vi "Optical Beacon - Hazardous Area Standard.vi"() -> ()   [LabVIEW 2015]
uses:
  <vilib>/userdefined/High Color/IMAQdx.ctl
  <vilib>/vision/driver/NI_Vision_Acquisition_Software.lvlib
  <vilib>/vision/NI_Vision_Development_Module.lvlib
  <resource>/objmgr/imaqdx.rc
panel:
  in  "Stop 2":bool
  out "Optical Beacon":bool
  out "Color Spectrum 4":dbl[](array[numeric]) format="%.2f"
  in  "Color Sensitivity 4":u32(ring) items=["Low", "Medium", "High"]
  out "Image 4":T1(plugin-control)
  out "Color Spectrum 3":dbl[](array[numeric]) format="%.2f"
  in  "Color Sensitivity 3":u32(ring) items=["Low", "Medium", "High"]
  out "Image 3":T1(plugin-control)
  out "Y Resoloution":i32
  out "X Resoloution":i32
  out "Video Modes":string
  in  "Video Mode":dbl min=0.0 max=5.0 step=1.0
  in  "Camera":T2
  in  "Stop":bool
  out "Image 1":T1(plugin-control)
  in  "Color Sensitivity 1":u32(ring) items=["Low", "Medium", "High"]
  out "Color Spectrum 1":dbl[](array[numeric]) format="%.2f"
  out "YELLOW Close":bool
  out "YELLOW Detect":bool
  out "RED Close":bool
  out "RED Detect":bool
  out "Hazardous Area":bool
  out "Image 2":T1(plugin-control)
  in  "Color Sensitivity 2":u32(ring) items=["Low", "Medium", "High"]
  out "Color Spectrum 2":dbl[](array[numeric]) format="%.2f"
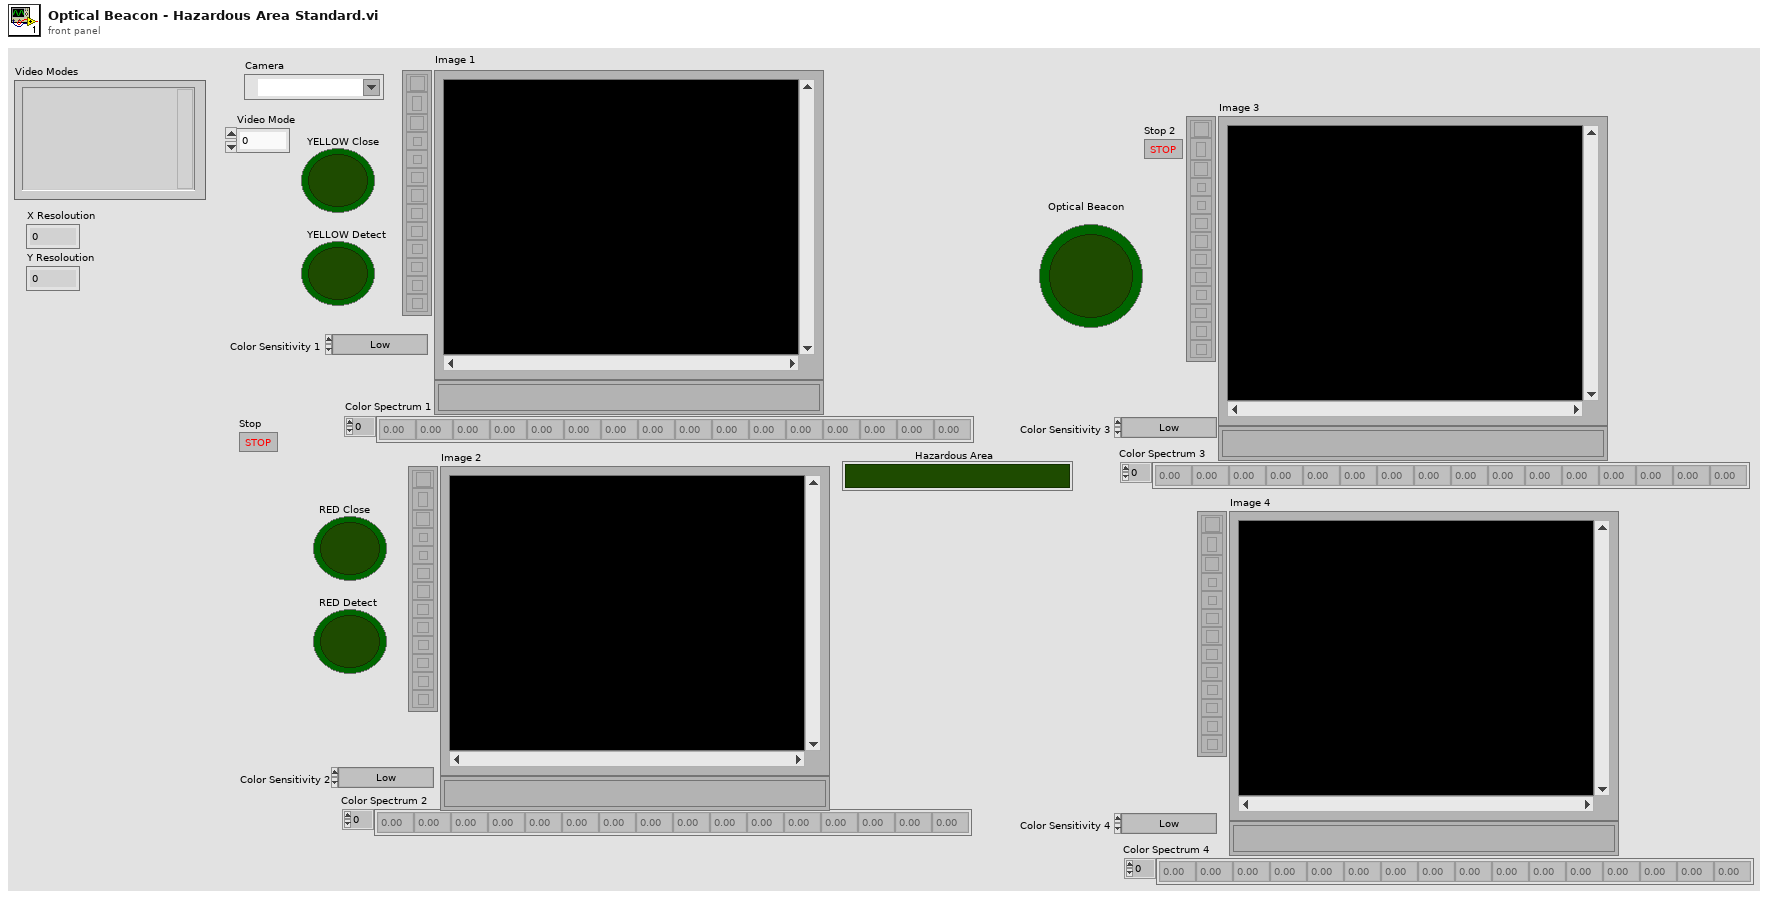
[diagram p1: front panel]
types:
  T1 = typedef "IMAQ Image.ctl" = refnum<image>
  T2 = typedef "IMAQdx.ctl" = refnum<k21>
  T3 = cluster{"Global Rectangle":i32[], "Contours":cluster{"Contour Type":u32, "ROI Type":u32, "Points":i32[]}[]}
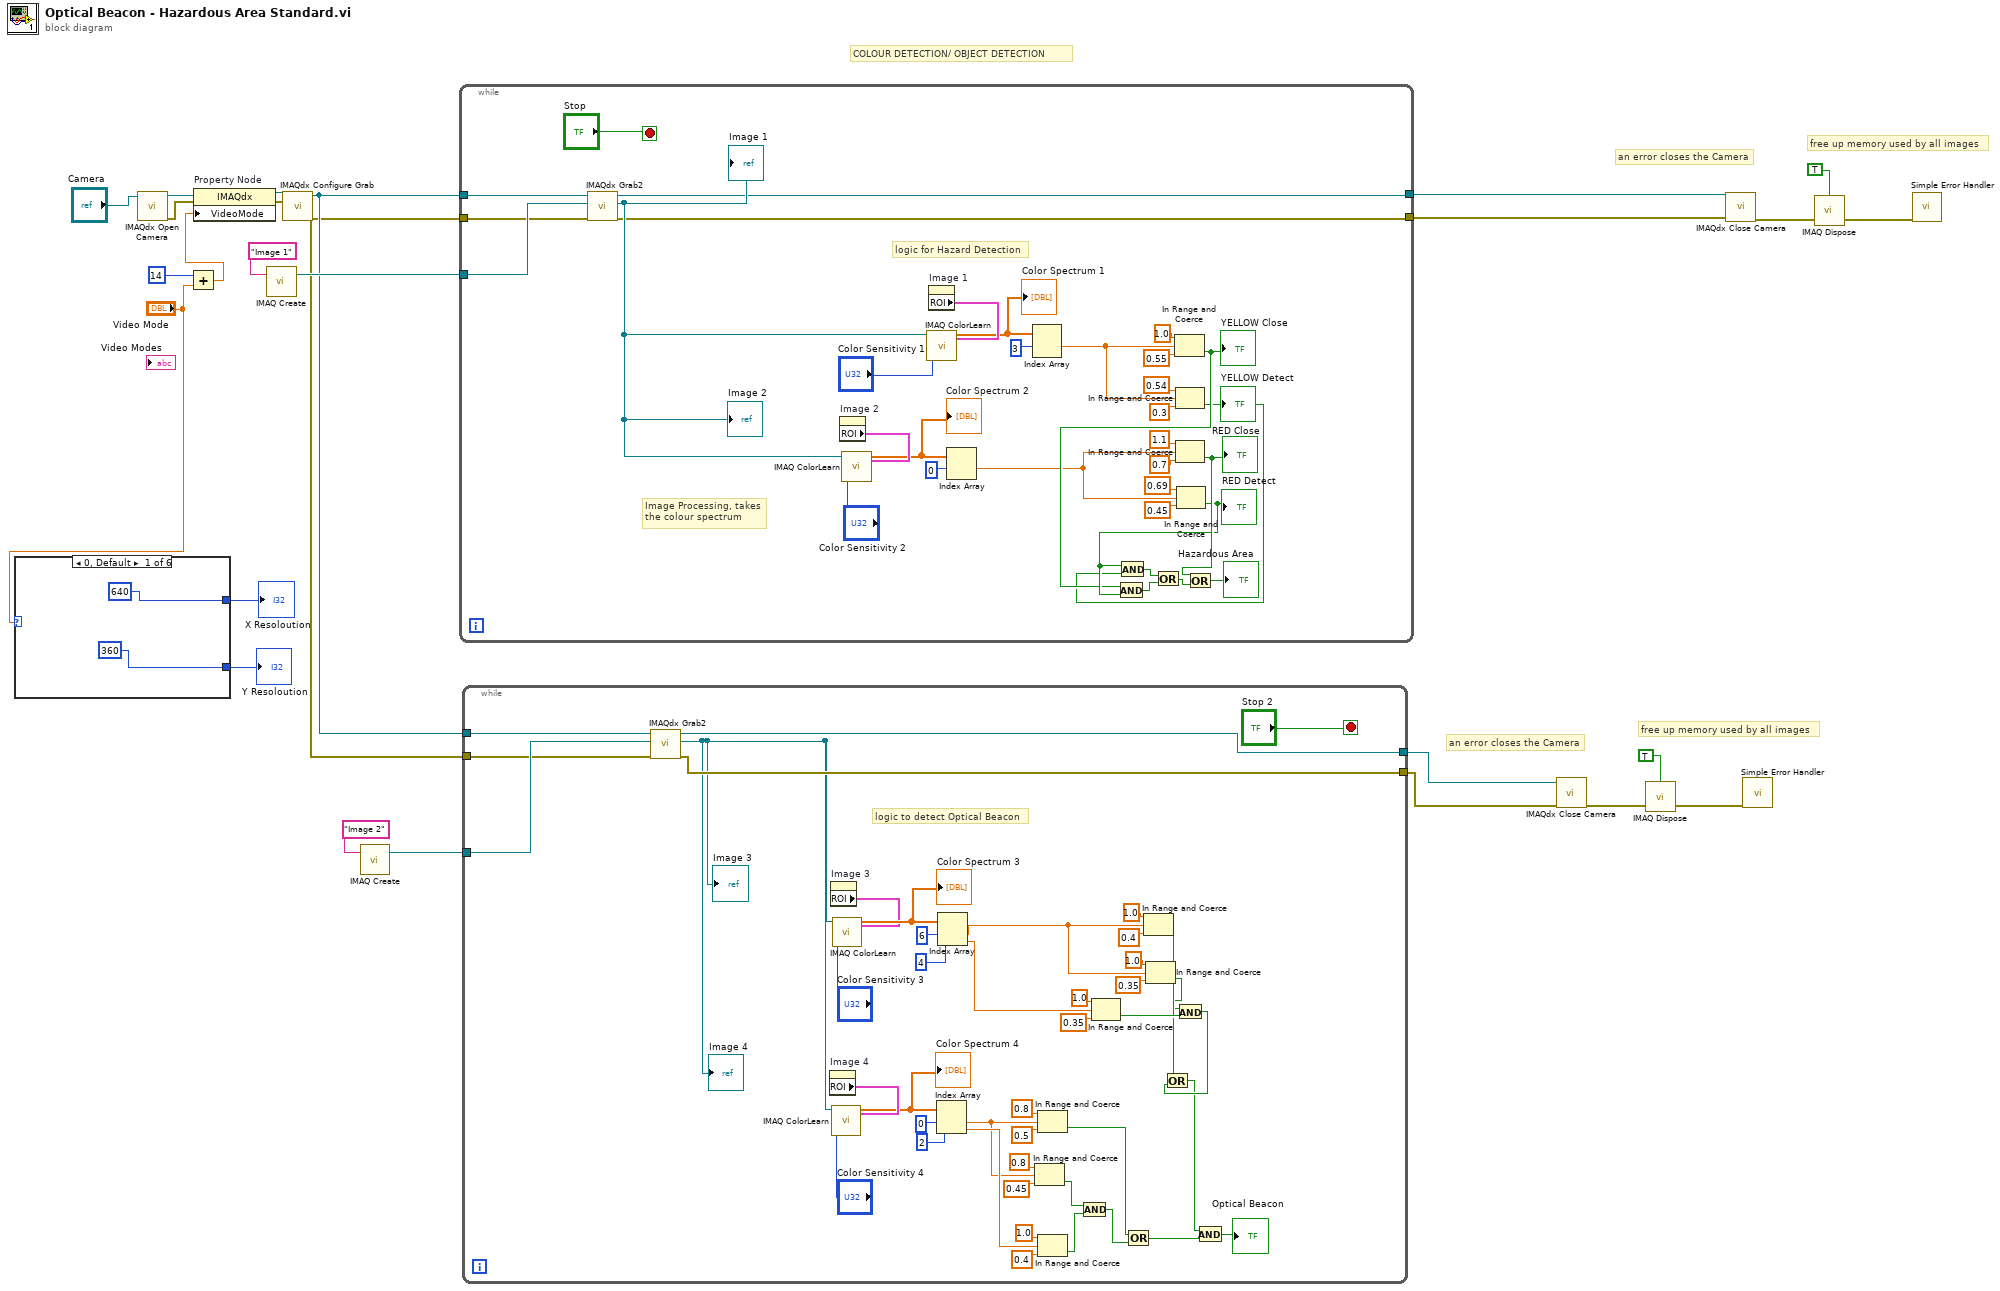
[diagram p0: block diagram]
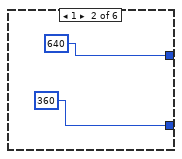
[diagram p2: hidden frame]
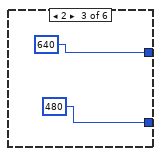
[diagram p3: hidden frame]
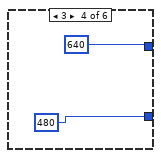
[diagram p4: hidden frame]
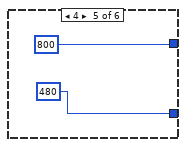
[diagram p5: hidden frame]
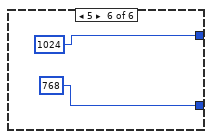
[diagram p6: hidden frame]
diagram:
  # "an error closes the Camera"
  # "free up memory used by all images"
  # "COLOUR DETECTION/ OBJECT DETECTION"
  # "an error closes the Camera"
  # "free up memory used by all images"
  n1 = case shown="0, Default" "Video Mode" {
    tunnel: [640 640 640 640 800 1024] -> w11
    tunnel: [360 360 480 480 480 768] -> w10
    frame 0, Default {
    }
    frame 1 {
    }
    frame 2 {
    }
    frame 3 {
    }
    frame 4 {
    }
    frame 5 {
    }
  }
  "X Resoloution" <- w11
  "Y Resoloution" <- w10
  n2 = call <vilib>:"IMAQdx Open Camera.vi"("Session In"="Camera") -> ("error out"=w23:errorcluster, "Session Out"=w24:T2)  [unwired: 9 in]
  n3 = Add(x=14, y="Video Mode") -> (x+y=w14:dbl)
  n4 = property on="Property Node" class="IMAQdx"(reference=w24, error in=w23, "VideoMode"=w14) -> (reference out=w22:T2, error out=w21:errorcluster)
  n5 = call "IMAQ Create"("Image Name"="Image 1") -> ("New Image"=w25:T1)  [unwired: 4 in, 1 out]
  n6 = call <vilib>:"IMAQdx Configure Grab.vi"("error in"=w21, "Session In"=w22) -> ("error out"=w1:errorcluster, "Session Out"=w2:T2)  [unwired: 8 in]
  n7 = call "IMAQ Create"("Image Name"="Image 2") -> ("New Image"=w3:T1)  [unwired: 4 in, 1 out]
  n8 = while {
    tunnel: w2 -> [w70]
    tunnel: w1 -> [w42]
    tunnel: [w39] -> w13
    tunnel: [w40] -> w19
    tunnel: w25 -> [w69]
    stop <- "Stop" stop-if-true
    # "Image Processing, takes\nthe colour spectrum"
    # "logic for Hazard Detection"
    n9 = call <vilib>:"IMAQdx Grab2.vi"("error in"=w42, "Image In"=w69, "Session In"=w70) -> ("error out"=w40:errorcluster, "Image Out"=w41:T1, "Session Out"=w39:T2)  [unwired: 5 in, 1 out]
    "Image 1" <- w41
    "Image 2" <- w41
    n10 = property on="Image 2" class="ImageControl"() -> ("ROI"=w48:T3)  [unwired: 2 in, 2 out]
    n11 = call "IMAQ ColorLearn"("ROI Descriptor"=w48, "Image"=w41, "Color Sensitivity"="Color Sensitivity 2") -> ("Color Spectrum"=w43:dbl[])  [unwired: 5 in, 1 out]
    "Color Spectrum 2" <- w43
    n12 = property on="Image 1" class="ImageControl"() -> ("ROI"=w67:T3)  [unwired: 2 in, 2 out]
    n13 = call "IMAQ ColorLearn"("ROI Descriptor"=w67, "Image"=w41, "Color Sensitivity"="Color Sensitivity 1") -> ("Color Spectrum"=w66:dbl[])  [unwired: 5 in, 1 out]
    "Color Spectrum 1" <- w66
    n14 = Index Array(array=w43, index #1=0 ("index")) -> (element #1=w44:dbl)  [unwired: 1 in, 1 out]
    n15 = Index Array(array=w66, index #1=3 ("index")) -> (element #1=w57:dbl)  [unwired: 1 in, 1 out]
    n16 = In Range and Coerce(upper limit=1.0, x=w57, lower limit=0.55) -> (In Range?=w50:bool)  [unwired: 1 out]
    "YELLOW Close" <- w50
    n17 = In Range and Coerce(upper limit=0.54, x=w57, lower limit=0.3) -> (In Range?=w49:bool)  [unwired: 1 out]
    "YELLOW Detect" <- w49
    n18 = In Range and Coerce(upper limit=1.1, x=w44, lower limit=0.7) -> (In Range?=w56:bool)  [unwired: 1 out]
    "RED Close" <- w56
    n19 = In Range and Coerce(upper limit=0.69, x=w44, lower limit=0.45) -> (In Range?=w55:bool)  [unwired: 1 out]
    "RED Detect" <- w55
    n20 = And(x=w50, y=w55) -> (x .and. y?=w53:bool)
    n21 = And(x=w55, y=w49) -> (x .and. y?=w54:bool)
    n22 = Or(x=w54, y=w53) -> (x .or. y?=w52:bool)
    n23 = Or(x=w56, y=w52) -> (x .or. y?=→"Hazardous Area":bool)
  }
  n24 = while {
    tunnel: [w77] -> w6
    tunnel: [w76] -> w5
    tunnel: w3 -> [w74]
    tunnel: w2 -> [w73]
    tunnel: w1 -> [w72]
    stop <- "Stop 2" stop-if-true
    # "logic to detect Optical Beacon"
    n25 = call <vilib>:"IMAQdx Grab2.vi"("error in"=w72, "Image In"=w74, "Session In"=w73) -> ("error out"=w76:errorcluster, "Image Out"=w75:T1, "Session Out"=w77:T2)  [unwired: 5 in, 1 out]
    "Image 3" <- w75
    "Image 4" <- w75
    n26 = property on="Image 4" class="ImageControl"() -> ("ROI"=w111:T3)  [unwired: 2 in, 2 out]
    n27 = property on="Image 3" class="ImageControl"() -> ("ROI"=w112:T3)  [unwired: 2 in, 2 out]
    n28 = call "IMAQ ColorLearn"("ROI Descriptor"=w111, "Image"=w75, "Color Sensitivity"="Color Sensitivity 4") -> ("Color Spectrum"=w108:dbl[])  [unwired: 5 in, 1 out]
    "Color Spectrum 4" <- w108
    n29 = call "IMAQ ColorLearn"("ROI Descriptor"=w112, "Image"=w75, "Color Sensitivity"="Color Sensitivity 3") -> ("Color Spectrum"=w115:dbl[])  [unwired: 5 in, 1 out]
    "Color Spectrum 3" <- w115
    n30 = Index Array(array=w108, index #1=0 ("index"), index #2=2 ("index")) -> (element #1=w91:dbl, element #2=w101:dbl)
    n31 = Index Array(array=w115, index #1=6 ("index"), index #2=4 ("index")) -> (element #1=w88:dbl, element #2=w96:dbl)
    n32 = In Range and Coerce(upper limit=0.8, x=w91, lower limit=0.45) -> (In Range?=w83:bool)  [unwired: 1 out]
    n33 = In Range and Coerce(upper limit=0.8, x=w91, lower limit=0.5) -> (In Range?=w84:bool)  [unwired: 1 out]
    n34 = In Range and Coerce(upper limit=1.0, x=w101, lower limit=0.4) -> (In Range?=w82:bool)  [unwired: 1 out]
    n35 = And(x=w83, y=w82) -> (x .and. y?=w81:bool)
    n36 = In Range and Coerce(upper limit=1.0, x=w96, lower limit=0.35) -> (In Range?=w95:bool)  [unwired: 1 out]
    n37 = Or(x=w84, y=w81) -> (x .or. y?=w80:bool)
    n38 = In Range and Coerce(upper limit=1.0, x=w88, lower limit=0.4) -> (In Range?=w87:bool)  [unwired: 1 out]
    n39 = In Range and Coerce(upper limit=1.0, x=w88, lower limit=0.35) -> (In Range?=w86:bool)  [unwired: 1 out]
    n40 = And(x=w86, y=w95) -> (x .and. y?=w85:bool)
    n41 = Or(x=w87, y=w85) -> (x .or. y?=w79:bool)
    n42 = And(x=w79, y=w80) -> (x .and. y?=→"Optical Beacon":bool)
  }
  n43 = call <vilib>:"IMAQdx Close Camera.vi"("error in"=w5, "Session In"=w6) -> ("error out"=w7:errorcluster)  [unwired: 9 in]
  n44 = call "IMAQ Dispose"("All Images? (No)"=TRUE, "error in (no error)"=w7) -> ("error out"=w8:errorcluster)  [unwired: 4 in]
  n45 = call <vilib>:"IMAQdx Close Camera.vi"("error in"=w19, "Session In"=w13) -> ("error out"=w16:errorcluster)  [unwired: 9 in]
  n46 = call <vilib>:"Simple Error Handler.vi"("error in (no error)"=w8) -> ()  [unwired: 4 in, 5 out]
  n47 = call "IMAQ Dispose"("All Images? (No)"=TRUE, "error in (no error)"=w16) -> ("error out"=w17:errorcluster)  [unwired: 4 in]
  n48 = call <vilib>:"Simple Error Handler.vi"("error in (no error)"=w17) -> ()  [unwired: 4 in, 5 out]
